vi "Viasala Indigo 520-String Data.vi"(8 "error in (no error)":errorcluster, 10 "Viasala Probe Number":u16, 11 "Viasala Data Input":T1) -> (0 "error out":errorcluster, 2 "Viasala Data":string[][](array[string]), 3 "Viasala Data Output":T1)   [LabVIEW 2023]
uses:
  Type Definitions/Viasala Indigo 520 Data.ctl
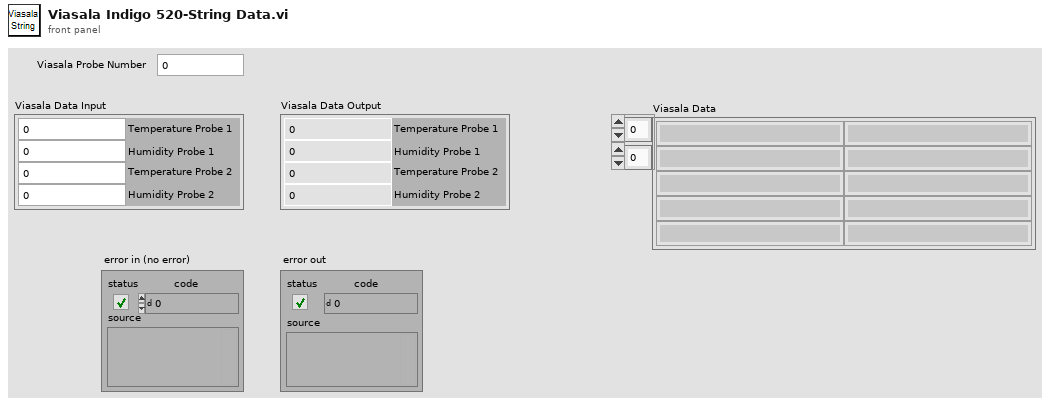
[diagram p1: front panel]
types:
  T1 = typedef "Viasala Indigo 520 Data.ctl" = cluster{"Temperature Probe 1":dbl, "Humidity Probe 1":dbl, "Temperature Probe 2":dbl, "Humidity Probe 2":dbl}
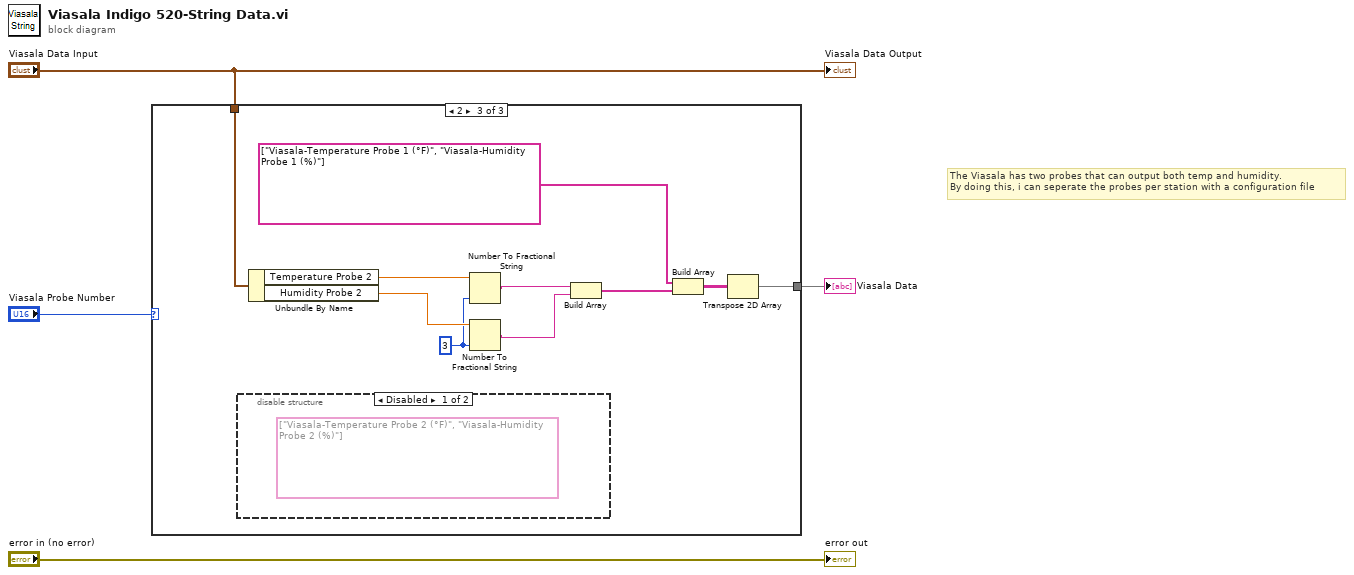
[diagram p0: block diagram]
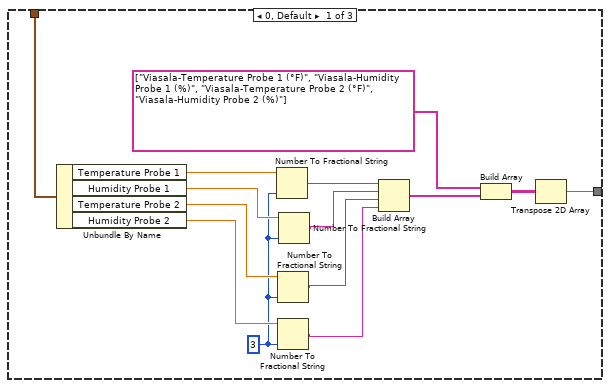
[diagram p2: hidden frame]
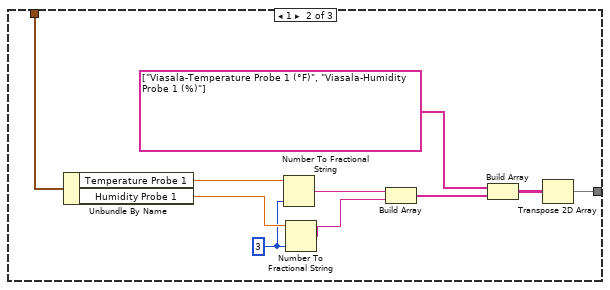
[diagram p3: hidden frame]
diagram:
  # "The Viasala has two probes that can output both temp and humidity. \nBy doing this, i can seperate the probes per station with a configuration file"
  n1 = case shown="2" "Viasala Probe Number" {
    tunnel: "Viasala Data Input" -> [w18 w21 w30]
    tunnel: [w5 w20 w31] -> w3
    frame 0, Default {
      w13 = i16 3 ("precision (6)")
      n2 = Unbundle By Name(w18) -> ("Temperature Probe 1"=w17:dbl, "Humidity Probe 1"=w16:dbl, "Temperature Probe 2"=w15:dbl, "Humidity Probe 2"=w14:dbl)
      n3 = Number To Fractional String(number=w17, precision (6)=w13) -> (F-format string=w12:string)  [unwired: 2 in]
      n4 = Number To Fractional String(number=w15, precision (6)=w13) -> (F-format string=w10:string)  [unwired: 2 in]
      n5 = Number To Fractional String(number=w14, precision (6)=w13) -> (F-format string=w9:string)  [unwired: 2 in]
      n6 = Number To Fractional String(number=w16, precision (6)=w13) -> (F-format string=w11:string)  [unwired: 2 in]
      n7 = Build Array(w12, w11, w10, w9) -> (w7:string[])
      n8 = Build Array(string[] ["Viasala-Temperature Probe 1 (°F)", "Viasala-Humidity Probe 1 (%)", "Viasala-Temperature Probe 2 (°F)", "Viasala-Humidity Probe 2 (%)"], w7) -> (w6:string[][])
      n9 = Transpose 2D Array(2D array=w6) -> (transposed array=w5:string[][])
    }
    frame 1 {
      w19 = i16 3 ("precision (6)")
      n10 = Unbundle By Name(w21) -> ("Temperature Probe 1"=w28:dbl, "Humidity Probe 1"=w27:dbl)
      n11 = Number To Fractional String(number=w28, precision (6)=w19) -> (F-format string=w26:string)  [unwired: 2 in]
      n12 = Number To Fractional String(number=w27, precision (6)=w19) -> (F-format string=w25:string)  [unwired: 2 in]
      n13 = Build Array(w26, w25) -> (w23:string[])
      n14 = Build Array(string[] ["Viasala-Temperature Probe 1 (°F)", "Viasala-Humidity Probe 1 (%)"], w23) -> (w22:string[][])
      n15 = Transpose 2D Array(2D array=w22) -> (transposed array=w20:string[][])
    }
    frame 2 {
      w32 = i16 3 ("precision (6)")
      n16 = disable-structure shown="Disabled" {
        frame Disabled {
          (unwired) string[] ["Viasala-Temperature Probe 2 (°F)", "Viasala-Humidity Probe 2 (%)"]
        }
        frame Enabled {
        }
      }
      n17 = Unbundle By Name(w30) -> ("Temperature Probe 2"=w38:dbl, "Humidity Probe 2"=w37:dbl)
      n18 = Number To Fractional String(number=w38, precision (6)=w32) -> (F-format string=w36:string)  [unwired: 2 in]
      n19 = Number To Fractional String(number=w37, precision (6)=w32) -> (F-format string=w35:string)  [unwired: 2 in]
      n20 = Build Array(w36, w35) -> (w34:string[])
      n21 = Build Array(string[] ["Viasala-Temperature Probe 1 (°F)", "Viasala-Humidity Probe 1 (%)"], w34) -> (w33:string[][])
      n22 = Transpose 2D Array(2D array=w33) -> (transposed array=w31:string[][])
    }
  }
  "Viasala Data" <- w3
  "Viasala Data Output" <- "Viasala Data Input"
  "error out" <- "error in (no error)"
